vi "FTW-Benchmark-Actors.vi"() -> ()   [LabVIEW 2013]
uses:
  Actor/src/Connector/FTW-ActorConnector.lvclass
panel:
  out "Actor Pool Spawn":dbl format="Actor Pool Spawn: %_3psec"
  out "Overall Pass?":bool
  out "Total Elapsed Time":dbl format="Messaging Time: %_3psec"
  out "\"FTW: Ping\" Times":cluster{dbl[]}[](graph)
  out "Results":T1(array[cluster])
  in  "Test to Perform":T2(radio)=enum."Parallel: 10x10"
  out "\"PING\" Times":cluster{dbl[]}[](graph)
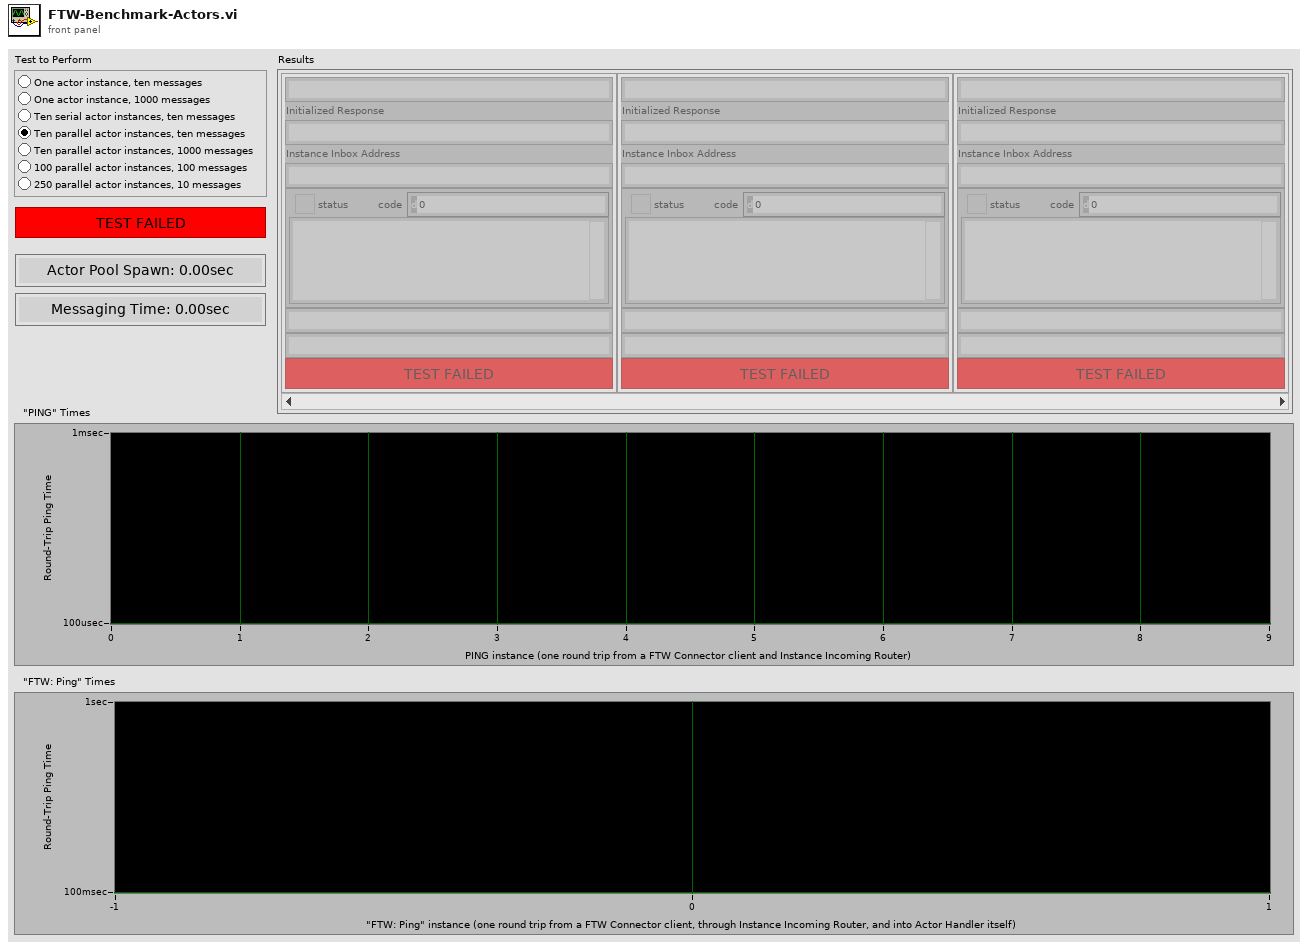
[diagram p1: front panel]
types:
  T1 = cluster{"Server Address":string, "Initialized Response":string, "Instance Inbox Address":string, "Error":errorcluster, "Server Address":string, "Server Address":string, "Pass?":bool}[]
  T2 = enum32{"Serial: 1x10", "Serial: 1x1000", "Serial: 10x10", "Parallel: 10x10", "Parallel: 10x100", "Parallel: 100x100", "Parallel: 250x10"}
  T3 = cluster{i32, "Initialized Response":string, "Instance Inbox Address":string, "Instance Publisher Address":string, "error out":errorcluster}
  T4 = cluster{i32, bool, bool, "Timed out?":bool, cluster{dbl[]}, cluster{dbl[]}, "error out":errorcluster}
  T5 = cluster{string, "Initialized Response":string, "Instance Inbox Address":string, "error out":errorcluster, string, string, bool}
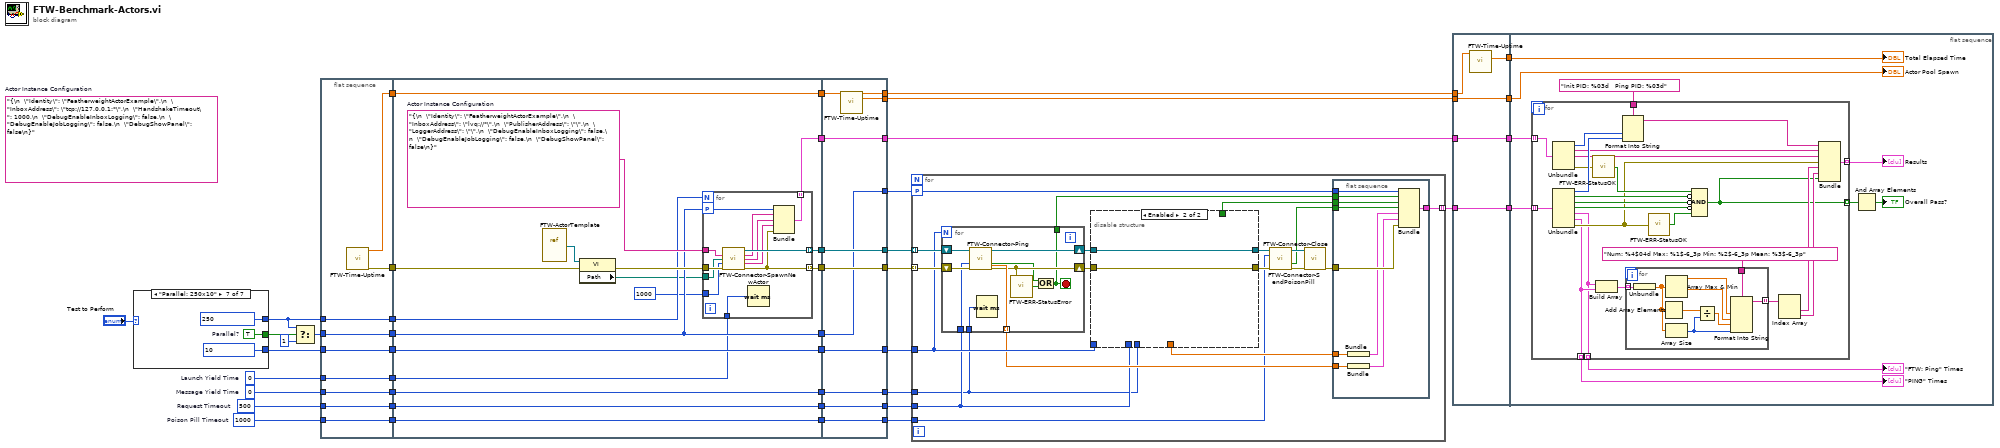
[diagram p0: block diagram]
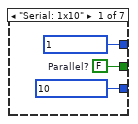
[diagram p2: hidden frame]
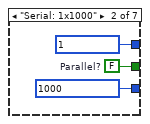
[diagram p3: hidden frame]
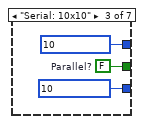
[diagram p4: hidden frame]
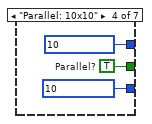
[diagram p5: hidden frame]
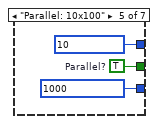
[diagram p6: hidden frame]
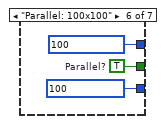
[diagram p7: hidden frame]
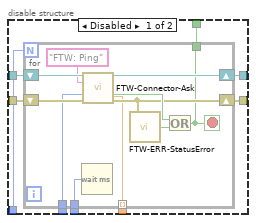
[diagram p8: hidden frame]
diagram:
  (unwired) "{\n  \"Identity\": \"FeatherweightActorExample\",\n  \"InboxAddress\": \"tcp://127.0.0.1:*\",\n  \"HandshakeTimeout\": 1000,\n  \"DebugEnableInboxLogging\": false,\n  \"DebugEnableJobLogging\": false,\n  \"DebugShowPanel\": false\n}"  # Actor Instance Configuration
  w1 = u32 0  # Message Yield Time
  w5 = u32 0  # Launch Yield Time
  w7 = 1000  # Poison Pill Timeout
  w9 = 500  # Request Timeout
  n1 = case shown="\"Parallel: 250x10\"" "Test to Perform" {
    tunnel: [1 1 10 10 10 100 250] -> w14
    tunnel: [10 1000 10 10 1000 100 10] -> w12
    tunnel: [w44 w47 w50 w53 w56 w59 w62] -> w18
    frame "Serial: 1x10" {
      w44 = FALSE  # Parallel?
    }
    frame "Serial: 1x1000" {
      w47 = FALSE  # Parallel?
    }
    frame "Serial: 10x10" {
      w50 = FALSE  # Parallel?
    }
    frame "Parallel: 10x10" {
      w53 = TRUE  # Parallel?
    }
    frame "Parallel: 10x100" {
      w56 = TRUE  # Parallel?
    }
    frame "Parallel: 100x100" {
      w59 = TRUE  # Parallel?
    }
    frame "Parallel: 250x10" {
      w62 = TRUE  # Parallel?
    }
  }
  n2 = Select(t=w14, s=w18, f=1) -> (s? t:f=w16:i32)
  n3 = flat-sequence {
    tunnel: [w73] -> w22
    tunnel: [w69] -> w21
    tunnel: [w72] -> w17
    tunnel: w16 -> [w72]
    tunnel: [w71] -> w15
    tunnel: w14 -> [w71]
    tunnel: [w70] -> w13
    tunnel: w12 -> [w70]
    tunnel: [w68] -> w10
    tunnel: w9 -> [w68]
    tunnel: [w67] -> w8
    tunnel: w7 -> [w67]
    tunnel: [w66] -> w6
    tunnel: w5 -> [w66]
    tunnel: [w65] -> w2
    tunnel: w1 -> [w65]
    tunnel: [w87] -> w34
    tunnel: [w86] -> w33
    tunnel: [w80] -> w32
    tunnel: [w82] -> w31
    tunnel: [w85] -> w30
    tunnel: [w83] -> w29
    tunnel: [w79] -> w25
    tunnel: [w78] -> w23
    tunnel: w22 -> [w84]
    tunnel: w21 -> [w83]
    tunnel: w17 -> [w82]
    tunnel: w15 -> [w81]
    tunnel: w13 -> [w80]
    tunnel: w10 -> [w79]
    tunnel: w8 -> [w78]
    tunnel: w6 -> [w77]
    tunnel: [w76] -> w3
    tunnel: w2 -> [w76]
    tunnel: [w109] -> w39
    tunnel: [w110] -> w40
    tunnel: [w111] -> w41
    tunnel: [w112] -> w42
    tunnel: [w113] -> w43
    tunnel: w34 -> [w113]
    tunnel: w33 -> [w112]
    tunnel: w32 -> [w111]
    tunnel: w31 -> [w110]
    tunnel: w30 -> [w109]
    tunnel: w29 -> [w108]
    tunnel: [w107] -> w27
    tunnel: [w106] -> w26
    tunnel: w25 -> [w106]
    tunnel: [w105] -> w24
    tunnel: w23 -> [w105]
    tunnel: [w104] -> w11
    tunnel: [w103] -> w4
    tunnel: w3 -> [w103]
    frame #0 {
      n4 = call "FTW-Time-Uptime.vi"() -> ("Current Uptime"=w69:dbl, "error out"=w73:errorcluster)  [unwired: 13 in, 1 out]
    }
    frame #1 {
      w89 = "{\n  \"Identity\": \"FeatherweightActorExample\",\n  \"InboxAddress\": \"lvq://*\",\n  \"PublisherAddress\": \"\",\n  \"LoggerAddress\": \"\",\n  \"DebugEnableInboxLogging\": false,\n  \"DebugEnableJobLogging\": false,\n  \"DebugShowPanel\": false\n}"  # Actor Instance Configuration
      n5 = vi-ref "FTW-ActorTemplate.vi"() -> (w90:refnum<vi>)
      n6 = property class="VI"(reference=w90, error in=w84) -> (error out=w88:errorcluster, "Path"=w75:path)  [unwired: 1 out]
      n7 = for {
        N: w81 -> [_]
        tunnel: w89 -> [w94]
        tunnel: w88 -> [w102]
        tunnel: [w101] -> w87 mode=indexing
        tunnel: [w96] -> w86 mode=indexing
        tunnel: [w97] -> w85 mode=indexing
        workers-P: w82 -> [w95]
        tunnel: w77 -> [w93]
        tunnel: w75 -> [w92]
        tunnel: 1000 -> [w91]
        n8 = call "FTW-Connector-SpawnNewActor.vi"("Configuration"=w94, "Actor VI Filepath"=w92, "Timeout"=w91, "error in"=w102) -> ("FTW Actor Connector"=w101:refnum<class "FTW-ActorConnector.lvclass">, "Initialized Response"=w100:string, "Instance Inbox Address"=w99:string, "Instance Publisher Address"=w98:string, "error out"=w96:errorcluster)  [unwired: 7 in]
        n9 = Wait (ms)(milliseconds to wait=w93) -> ()  [unwired: 1 out]
        n10 = Bundle(w95, "Initialized Response"=w100, "Instance Inbox Address"=w99, "Instance Publisher Address"=w98, "error out"=w96) -> (w97:T3)  [unwired: 1 in]
      }
    }
    frame #2 {
      n11 = call "FTW-Time-Uptime.vi"("Previous Uptime"=w108) -> ("Current Uptime"=w104:dbl, "Elapsed Time"=w107:dbl)  [unwired: 12 in, 1 out]
    }
  }
  n12 = for {
    tunnel: w43 -> [w131] mode=indexing
    tunnel: w42 -> [w130] mode=indexing
    tunnel: w41 -> [w125]
    workers-P: w40 -> [w124]
    tunnel: [w121] -> w38 mode=indexing
    tunnel: w26 -> [w117]
    tunnel: w24 -> [w116]
    tunnel: w4 -> [w115]
    n13 = for {
      N: w125 -> [_]
      tunnel: [w162] -> w118 mode=indexing
      shift-right: [w163] -> w129
      shift-left: w131 -> [w165]
      shift-right: [w161] -> w128
      shift-left: w130 -> [w164]
      tunnel: [w158] -> w123
      tunnel: w117 -> [w157]
      tunnel: w115 -> [w156]
      stop <- w158 stop-if-true
      n14 = call "FTW-Connector-Ping.vi"("FTW Actor Connector"=w165, "Timeout"=w157, "error in"=w164) -> ("FTW Actor Connector out"=w163:refnum<class "FTW-ActorConnector.lvclass">, "Timed out?"=w159:bool, "Roundtrip Time"=w162:dbl, "error out"=w161:errorcluster)  [unwired: 8 in, 1 out]
      n15 = Wait (ms)(milliseconds to wait=w156) -> ()  [unwired: 1 out]
      n16 = call "FTW-ERR-StatusError.vi"("error to check"=w161) -> ("Error?"=w160:bool)
      n17 = Or(x=w159, y=w160) -> (x .or. y?=w158:bool)
    }
    n18 = disable-structure shown="Enabled" {
      disable-tunnel: w129 -> [w142 w155]
      disable-tunnel: w128 -> [w141 w154]
      disable-tunnel: [w140 w155] -> w127
      disable-tunnel: [w139 w154] -> w126
      disable-tunnel: w125 -> [w138 _]
      disable-tunnel: [w137 _] -> w122
      disable-tunnel: [w136 _] -> w119
      disable-tunnel: w117 -> [w135 _]
      disable-tunnel: w115 -> [w134 _]
      frame Disabled {
        n19 = for {
          N: w138 -> [_]
          tunnel: [w148] -> w136 mode=indexing
          shift-right: [w151] -> w140
          shift-left: w142 -> [w152]
          shift-right: [w149] -> w139
          shift-left: w141 -> [w147]
          tunnel: [w146] -> w137
          tunnel: w135 -> [w145]
          tunnel: w134 -> [w144]
          stop <- w146 stop-if-true
          n20 = Wait (ms)(milliseconds to wait=w144) -> ()  [unwired: 1 out]
          n21 = call "FTW-Connector-Ask.vi"("FTW Actor Connector"=w152, "Request Header"="FTW: Ping", "Timeout"=w145, "error in"=w147) -> ("FTW Actor Connector out"=w151:refnum<class "FTW-ActorConnector.lvclass">, "Timed out?"=w150:bool, "Roundtrip Time"=w148:dbl, "error out"=w149:errorcluster)  [unwired: 6 in, 2 out]
          n22 = call "FTW-ERR-StatusError.vi"("error to check"=w149) -> ("Error?"=w153:bool)
          n23 = Or(x=w150, y=w153) -> (x .or. y?=w146:bool)
        }
      }
      frame Enabled {
      }
    }
    n24 = call-dynamic "FTW-Connector-SendPoisonPill.vi"("FTW Actor Connector"=w127, "Timeout"=w116, "error in"=w126) -> ("FTW Actor Connector out"=w133:refnum<class "FTW-ActorConnector.lvclass">, "Timed out?"=w114:bool, "error out"=w132:errorcluster)  [unwired: 8 in, 2 out]
    n25 = call-dynamic "FTW-Connector-Close.vi"("FTW Actor Connector"=w133, "error in"=w132) -> ("error out"=w120:errorcluster)  [unwired: 13 in]
    n26 = flat-sequence {
      tunnel: w124 -> [w175]
      tunnel: w123 -> [w174]
      tunnel: w122 -> [w173]
      tunnel: [w172] -> w121
      tunnel: w114 -> [w171]
      tunnel: w120 -> [w170]
      tunnel: w119 -> [w168]
      tunnel: w118 -> [w166]
      frame #0 {
        n27 = Bundle(w168) -> (w169:cluster{dbl[]})  [unwired: 1 in]
        n28 = Bundle(w166) -> (w167:cluster{dbl[]})  [unwired: 1 in]
        n29 = Bundle(w175, w174, w173, "Timed out?"=w171, w169, w167, "error out"=w170) -> (w172:T4)  [unwired: 1 in]
      }
    }
  }
  n30 = flat-sequence {
    tunnel: w38 -> [w179]
    tunnel: w39 -> [w180]
    tunnel: [w180] -> w37
    tunnel: [w179] -> w36
    tunnel: [w178] -> w35
    tunnel: [w177] -> w28
    tunnel: w27 -> [w177]
    tunnel: w11 -> [w176]
    tunnel: w37 -> [w190]
    tunnel: w36 -> [w189]
    tunnel: w35 -> [w184]
    tunnel: w28 -> [w181]
    frame #0 {
      n31 = call "FTW-Time-Uptime.vi"("Previous Uptime"=w176) -> ("Elapsed Time"=w178:dbl)  [unwired: 12 in, 2 out]
    }
    frame #1 {
      n32 = for {
        tunnel: w190 -> [w214] mode=indexing
        tunnel: w189 -> [w213] mode=indexing
        tunnel: "Init PID: %03d   Ping PID: %03d" ("format string") -> [w212]
        tunnel: [w195] -> w187 mode=indexing
        tunnel: [w191] -> w186 mode=indexing
        tunnel: [w194] -> w185 mode=indexing
        tunnel: [w193] -> w183 mode=indexing
        n33 = Unbundle(w214) -> (w211:i32, "Initialized Response"=w202:string, "Instance Inbox Address"=w201:string, "error out"=w209:errorcluster)  [unwired: 1 out]
        n34 = Unbundle(w213) -> (w210:i32, w207:bool, w206:bool, "Timed out?"=w205:bool, w191:cluster{dbl[]}, w194:cluster{dbl[]}, "error out"=w200:errorcluster)
        n35 = call "FTW-ERR-StatusOK.vi"("error to check"=w209) -> ("Status OK?"=w208:bool)
        n36 = Build Array(w191, w194) -> (w199:cluster{dbl[]}[])
        n37 = Format Into String(format string=w212, w211, w210) -> (resulting string=w203:string)  [unwired: 2 in, 1 out]
        n38 = for {
          tunnel: w199 -> [w219] mode=indexing
          tunnel: [w217] -> w198 mode=indexing
          tunnel: "Num: %4$04d Max: %1$-6_3p Min: %2$-6_3p Mean: %3$-6_3p" ("format string") -> [w216]
          n39 = Unbundle(w219) -> (w218:dbl[])
          n40 = Add Array Elements(numeric array=w218) -> (sum=w223:dbl)
          n41 = Array Max & Min(array=w218) -> (max value=w222:dbl, min value=w221:dbl)  [unwired: 2 out]
          n42 = Array Size(array=w218) -> (size(s)=w215:i32)
          n43 = Divide(x=w223, y=w215) -> (x/y=w220:dbl)
          n44 = Format Into String(format string=w216, w222, w221, w220, w215) -> (resulting string=w217:string)  [unwired: 2 in, 1 out]
        }
        n45 = call "FTW-ERR-StatusOK.vi"("error to check"=w200) -> ("Status OK?"=w204:bool)
        n46 = Compound Arithmetic op=AND(w208, invert w207, invert w206, invert w205, w204) -> (w193:bool)
        n47 = Index Array(array=w198) -> (element #1=w197:string, element #2=w196:string)  [unwired: 2 in]
        n48 = Bundle(w203, "Initialized Response"=w202, "Instance Inbox Address"=w201, "error out"=w200, w197, w196, w193) -> (w195:T5)  [unwired: 1 in]
      }
      "\"PING\" Times" <- w185
      "Results" <- w187
      "\"FTW: Ping\" Times" <- w186
      n49 = And Array Elements(Boolean array=w183) -> (logical AND=→"Overall Pass?":bool)
      "Total Elapsed Time" <- w184
      "Actor Pool Spawn" <- w181
    }
  }
